vi "bgk_3475_read.vi"(8 "error in (no error)":errorcluster caption="错误输入（无错误）", 9 "Last Data Array":dbl[](array[numeric])=[nan, nan, nan, nan] caption="原数据数组", 10 "unit adress array":string[](array[string])=["\u0001", "\u0003", "\u0004", "\u0005"] caption="设备地址数组", 11 "VISA Ref Input":refnum<visa-resource-name>="COM2" caption="VISA引用句柄输入") -> (0 "error out":errorcluster caption="错误输出", 1 "New Data Array":dbl[](array[numeric]) caption="新数据数组", 3 "VISA Ref Output":refnum<visa-resource-name> caption="VISA引用句柄输出")   [LabVIEW 2015]
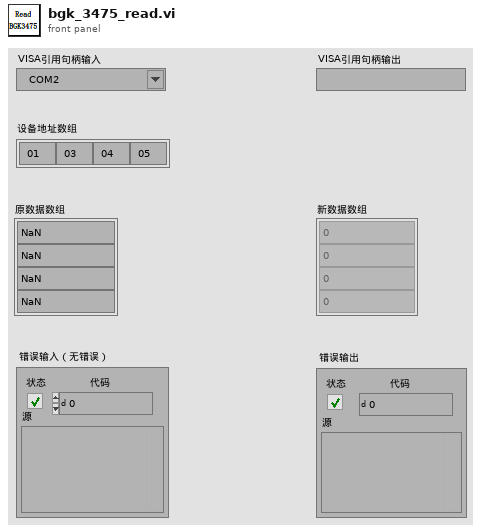
[diagram p1: front panel]
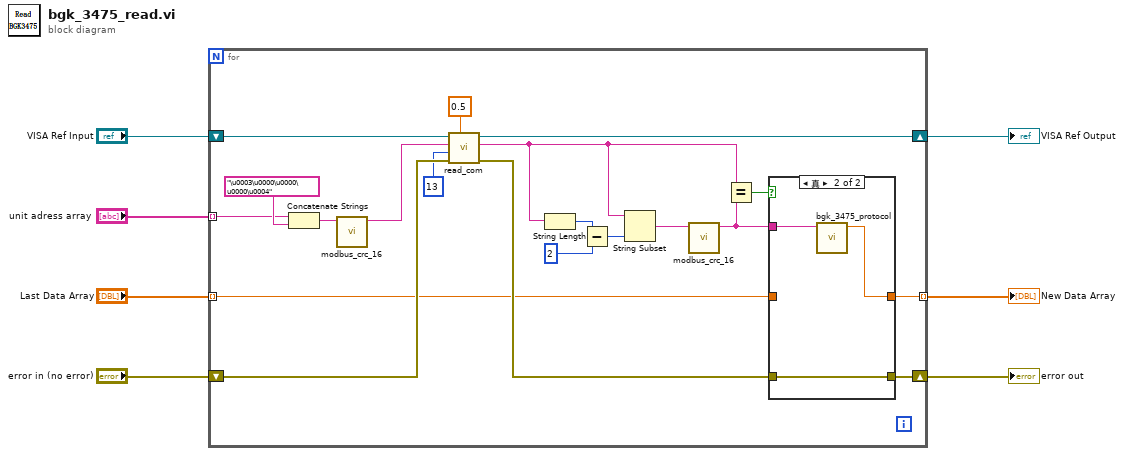
[diagram p0: block diagram]
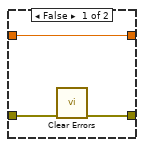
[diagram p2: hidden frame]
diagram:
  n1 = for {
    tunnel: "unit adress array" -> [w17] mode=indexing
    shift-right: [w27] -> w7
    shift-left: "VISA Ref Input" -> [w26]
    shift-right: [w23] -> w4
    shift-left: "error in (no error)" -> [w25]
    tunnel: "Last Data Array" -> [w21] mode=indexing
    tunnel: [w20] -> w1 mode=indexing
    n2 = Concatenate Strings(w17, "\u0003\u0000\u0000\u0000\u0004" ("数据发送区")) -> (w18:string)
    n3 = call "modbus_crc_16.vi"("String"=w18) -> ("String & CRC-16"=w16:string)  [unwired: 9 in, 1 out]
    n4 = call "read_com.vi"("wait sec"=0.5, "error in"=w25, "read bytes"=u32 13, "write to buffer"=w16, "VISA resource name in"=w26) -> ("error out"=w22:errorcluster, "read from buffer"=w11:string, "VISA resource name out"=w27:refnum<visa-resource-name>)  [unwired: 3 in, 1 out]
    n5 = String Length(string=w11) -> (length=w14:i32)
    n6 = Subtract(x=w14, y=2) -> (x-y=w13:i32)
    n7 = String Subset(string=w11, length (rest)=w13) -> (substring=w15:string)  [unwired: 1 in]
    n8 = call "modbus_crc_16.vi"("String"=w15) -> ("String & CRC-16"=w9:string)  [unwired: 9 in, 1 out]
    n9 = Equal?(x=w11, y=w9) -> (x = y?=w10:bool)
    n10 = case shown="真" w10 {
      tunnel: w9 -> [_ w32]
      tunnel: w22 -> [w30 w33]
      tunnel: [w29 w33] -> w23
      tunnel: w21 -> [w28 _]
      tunnel: [w28 w31] -> w20
      frame False {
        n11 = call <vilib>:"Clear Errors.vi"("error in (no error)"=w30) -> ("error out"=w29:errorcluster)  [unwired: 5 in, 1 out]
      }
      frame True {
        n12 = call "bgk_3475_protocol.vi"("read from buffer"=w32) -> ("data"=w31:sgl)  [unwired: 10 in]
      }
    }
  }
  "New Data Array" <- w1
  "VISA Ref Output" <- w7
  "error out" <- w4
